vi "GetBold.vi"(8 "error in (no error)":errorcluster, 11 "Font in":refnum<class "Font.lvclass">) -> (0 "error out":errorcluster, 2 "Bold?":bool, 3 "Font out":refnum<class "Font.lvclass">)   [LabVIEW 2021, in "Picture2D.lvlib" / "Font.lvclass"]
uses:
  Font.lvclass
  Font.lvclass/Font.ctl
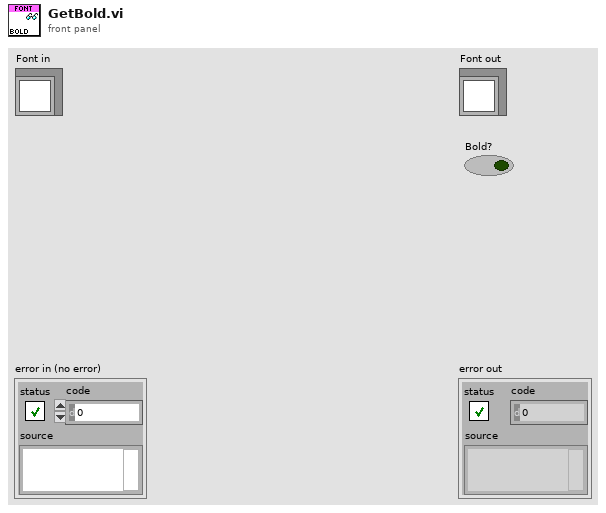
[diagram p1: front panel]
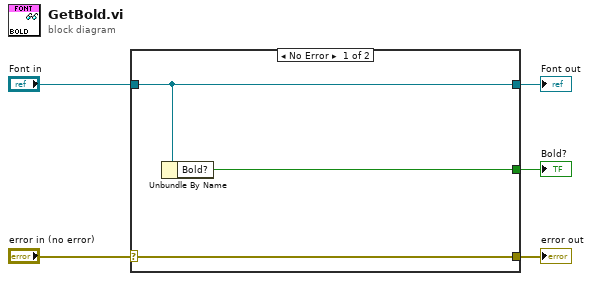
[diagram p0: block diagram]
diagram:
  n1 = case shown="No Error" "error in (no error)" {
    selector: "error in (no error)" -> [w8 w9]
    tunnel: [w8 w9] -> w4
    tunnel: [w7 w10] -> w2
    tunnel: "Font in" -> [w7 w10]
    tunnel: [w6 _] -> w1
    frame No Error {
      n2 = Unbundle By Name(w7) -> ("Bold?"=w6:bool)
    }
    frame Error {
    }
  }
  "error out" <- w4
  "Font out" <- w2
  "Bold?" <- w1
